vi "Careful_approach.vi"(8 "Error in (no error)":errorcluster, 11 "Application ref in":refnum<vi>) -> (0 "Error out":errorcluster, 1 "steps_taken":i32, 2 "approached?":bool, 3 "Application ref out":refnum<vi>)   [LabVIEW 2019]
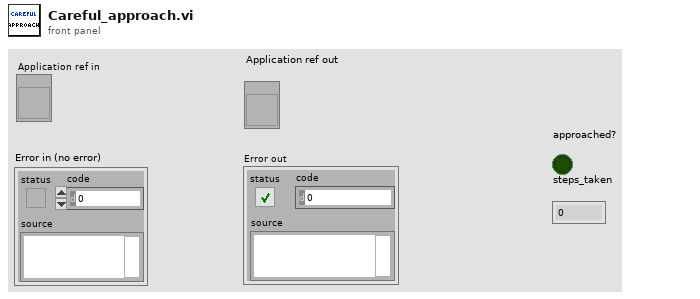
[diagram p1: front panel]
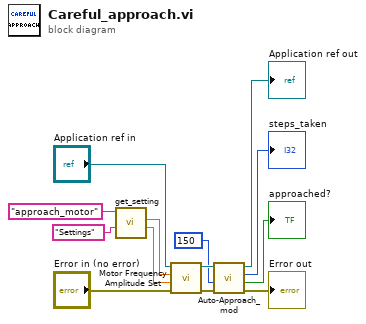
[diagram p0: block diagram]
diagram:
  n1 = call "get_setting.vi"("section"="Settings", "key"="approach_motor") -> ("output 2"=w10:dbl, "output 1"=w11:dbl)  [unwired: 5 in, 3 out]
  n2 = call <userlib>:"Motor Frequency Amplitude Set.vi"("Error in (no error)"="Error in (no error)", "Amplitude (V) (NaN=no change)"=w10, "Frequency (Hz) (NaN=no change)"=w11, "Application ref in"="Application ref in") -> ("Error out"=w6:errorcluster, "Application ref out"=w7:refnum<vi>)  [unwired: 6 in]
  n3 = call "Auto-Approach_mod.vi"("Error in"=w6, "max steps"=150, "Application reference"=w7) -> ("error out"=→"Error out":errorcluster, "Surface reached"=→"approached?":bool, "steps taken"=→"steps_taken":i32, "Application ref out"=→"Application ref out":refnum<vi>)  [unwired: 3 in]
